vi "Write Data Model.vi"(8 "error in (no error)":errorcluster, 10 "Data Model":refnum<class "Device Data Model.lvclass">, 11 "Master CR in":refnum<class "WebSocket Client CR.lvclass">) -> (0 "error out":errorcluster, 3 "Master CR out":refnum<class "WebSocket Client CR.lvclass">)   [LabVIEW 2021, in "WebSockets.lvlib" / "WebSocket Client CR.lvclass"]
uses:
  WebSocket Client CR.lvclass
  Modbus_v121c/Data Model/Device Data Model.lvclass
  WebSocket Client CR.lvclass/WebSocket Client CR.ctl
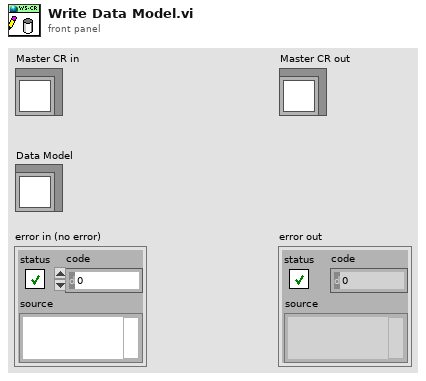
[diagram p1: front panel]
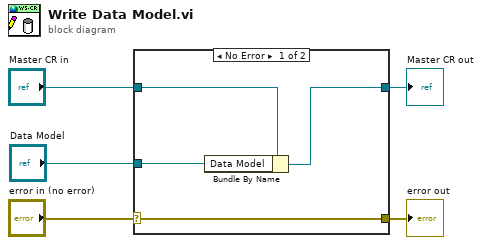
[diagram p0: block diagram]
diagram:
  n1 = case shown="No Error" "error in (no error)" {
    selector: "error in (no error)" -> [w7 w10]
    tunnel: [w7 w10] -> w4
    tunnel: [w8 w11] -> w2
    tunnel: "Master CR in" -> [w9 w11]
    tunnel: "Data Model" -> [w6 _]
    frame No Error {
      n2 = Bundle By Name(cluster=w9, "Data Model"=w6) -> (w8:refnum<class "WebSocket Client CR.lvclass">)
    }
    frame Error {
    }
  }
  "error out" <- w4
  "Master CR out" <- w2
